vi "UHR-Fleezers Control (host) - 10.4.vi"() -> ()   [LabVIEW 2011] (continued)
  T12 = cluster{"output high":fxp<+/-,16,1>, "output low":fxp<+/-,16,1>}
  T13 = cluster{"Set 1":fxp<+/-,16,1>, "Set 2":fxp<+/-,16,1>}
  T14 = cluster{"proportional gain (Kc)":i16, "integral gain (Kc*Ts/Ti)":i16, "derivative gain (Kc*Td/Ts)":i16}
  T15 = cluster{"Set 1":bool, "Set 2":bool, "Set 3":bool}
  T16 = typedef "LVMinMaxIncTypeDef.ctl" = cluster{"Minimum":dbl, "Maximum":dbl, "Increment":dbl}
  T17 = typedef "Image Type" = u32
  T18 = typedef "nirio_resource_hc.ctl" = tag
  T19 = typedef "openfpgaref.8.6.ctl" = refnum<k20>
  T20 = cluster{"New Image":T2, "New Image":T2, "New Image":T2, "New Image":T2}
  T21 = typedef "XDNodeRunTimeDep.lvlib/timing_clust.ctl" = cluster{"Expected End [f-1]":u64, "Actual End [f-1]":u64, "Finished Late? [f-1]":bool, "Expected End [i-1]":u64, "Actual End [i-1]":u64, "Finished Late? [i-1]":bool, "Expected Start [i]":u64, "Actual Start [i]":u64, "Expected Start [f]":u64, "Actual Start [f]":u64, "Source Name":string, "Structure Name":string, "Period":i64, "Deadline":i64, "Offset":i64, "Start":i64, "Priority":i32, "Timeout":i32, "Mode":T22, "Wakeup Reason":T23, "Error":errorcluster, "Source Type":string, "Secondary Source Type":string, "Global End Time":u64, "Global Start Time":u64, "Frame Duration":u64, "Iteration Duration":u64, "Assigned CPU":i32, "I/O Scan Engine Mode":u32}
  T22 = typedef "XDNodeRunTimeDep.lvlib/nitl_modes.ctl" = enum32{"No Change", "Process missed periods, maintain original phase", "Discard missed periods, maintain original phase", "Process missed periods, ignore original phase", "Discard missed periods, ignore original phase"}
  T23 = typedef "XDNodeRunTimeDep.lvlib/wakeup.ctl" = enum32{"Normal", "Aborted", "Asynchronous wakeup", "Timing source error", "Timed loop error", "Timeout"}
  T24 = enum16{"big-endian, network order", "native, host order", "little-endian"}
  T25 = enum16{"open", "replace", "create", "open or create", "replace or create", "replace or create with confirmation"}
  T26 = cluster{"Scan Range AOD (nm) 2":dbl, "Step Size AOD (nm) 2":dbl, "Scan Speed AOD (nm/s) 2":dbl, "Number of scans (AOD) 2":u16, "Label":string}
  T27 = cluster{"[0]":dbl, "[1]":dbl, "[2]":dbl, "[3]":dbl, "[4]":dbl, "[5]":dbl}
  T28 = cluster{"Diameter (mm)":dbl, "Units":dbl, "Volume":dbl, "Rate":dbl}
  T29 = cluster{"Left":i32, "Top":i32, "Width":u32, "Height":u32}
  T30 = cluster{cluster{"Left":i32, "Top":i32, "Width":u32, "Height":u32}}[]
  T31 = enum32{"setting", "request", "request control", "info", "statistics", "system settings", "I/O sub system", "HRT control", "camera descriptions", "device specific data", "event sub system settings", "event sub system results", "image memory manager"}
  T32 = typedef "AviRefnum.ctl" = refnum<k1>
  T33 = typedef "imagedata.ctl" = cluster{"image type":i32, "image depth":i32, "image":u8[], "mask":u8[], "colors":u32[], "Rectangle":cluster{"left":i16, "top":i16, "right":i16, "bottom":i16}}
  T34 = enum32{"Normal Display", "Dual Display (APD)", "FFT", "High Res Display"}
  T35 = cluster{"Origin Pixel":cluster{"X":sgl, "Y":sgl}, "Angle Relative to Horizontal (deg)":sgl, "Axis Reference":u32}
  T36 = typedef "Simple Grid Descriptor" = cluster{"X Step":sgl, "Y Step":sgl, "Unit":T37}
  T37 = typedef "Image Unit" = enum32{"Undefined", "Angström", "Micrometer", "Millimeter", "Centimeter", "Meter", "Kilometer", "Microinch", "Inch", "Feet", "Nautical miles", "Standard miles", "Steps"}
  T38 = cluster{"averaging mode":u16, "weighting mode":u16, "number of averages":u32}
  T39 = cluster{"dB On (F)":bool, "unwrap phase (F)":bool, "convert to degree (F)":bool}
  T40 = cluster{string, string, string, string, string, string, string, string}
  T41 = cluster{string, string, string, string, string, string, string, string, string, string, string, string}
  T42 = cluster{string, string, string, string, string, string, string, string, string, string, string, string, string}
  T43 = cluster{string, string, string, string, string, string, string, string, string, string, string, string, string, string}
  T44 = cluster{"BD 1 Frequency 1 (MHz)":dbl, "BD 1 Frequency 2 (MHz)":dbl}
  T45 = cluster{"f0":dbl, "df":dbl, "magnitude":dbl[]}[][]
  T46 = cluster{"Green FB Ch 0":i16, "Green FB Ch 1":i16, "Green FB Ch 2":i16}
  T47 = cluster{"Green FB Ch 0":dbl, "Green FB Ch 1":dbl, "Green FB Ch 2":dbl}
diagram:
  w55 = u16 20 items=["1.0"=10, "1.5"=15, "2.0"=20] ("stop bits (10: 1 bit)")
  w62 = T17 2 items=["Grayscale (U8)", "Grayscale (I16)", "Grayscale (SGL)", "Complex (CSG)", "RGB (U32)", "HSL (U32)", "RGB (U64)", "Grayscale (U16)"] ("Image Type")
  w125 = cluster{"output high":i16, "output low":i16} {"output high"=3000, "output low"=0} ("FB output range 1")
  w196 = 10.0 ("y")
  w195 = 32767.0 ("y")
  w211 = 6.0  # clock mult.
  w212 = 49152000.0  # TCXO frequ.
  n1 = Build Array("DIO count 1 (ticks)", "DIO count 2 (ticks)", "DIO count 3 (ticks)") -> (w112:u32[])
  n2 = local read "AO1"() -> (w190:dbl)
  n3 = local read "AO2"() -> (w189:dbl)
  n4 = local read "Scan Increment (MHz)"() -> (w207:dbl)
  n5 = local read "Continuous MCL Scanning"() -> (w177:bool)
  n6 = local read "Fast Scan Dir"() -> (w176:bool)
  n7 = local read "Number of scans (MCL)"() -> (w178:u64)
  n8 = property on="AI Count (ticks)" class="DigNum (strict)"("Val(Sgnl)"="AI Count (ticks)") -> ()  [unwired: 2 in, 2 out]
  n9 = Multiply(x=w190, y=w195) -> (x*y=w192:dbl)
  n10 = Multiply(x=w189, y=w195) -> (x*y=w194:dbl)
  n11 = Divide(x=w192, y=w196) -> (x/y=w191:dbl)
  n12 = Divide(x=w194, y=w196) -> (x/y=w193:dbl)
  n13 = To Word Integer(number=w191) -> (16bit integer=w188:i16)
  n14 = To Word Integer(number=w193) -> (16bit integer=w187:i16)
  n15 = Not(x=w176) -> (.not. x?=w171:bool)
  n16 = local read "Cycles/step (MCL)"() -> (w179:u64)
  n17 = Multiply(x=w207, y=1000.0) -> (x*y=w214:dbl)
  n18 = local read "Scan steps (MCL)"() -> (w180:u64)
  n19 = local write "Trap Pos FIFO Timeout"(u16 0 ("Trap Pos FIFO Timeout")) -> ()
  n20 = local read "Desired Scan Incr (V)"() -> (w182:dbl)
  n21 = Scale By Power Of 2(n=48, x=w214) -> (x*2^n=w215:dbl)
  n22 = Multiply(x=w212, y=w211) -> (x*y=w210:dbl)
  n23 = Divide(x=w215, y=w210) -> (x/y=w209:dbl)
  n24 = local read "Setpoints (V)"() -> (w228:cluster{"Set 1":dbl, "Set 2":dbl})
  n25 = To Quad Integer(1:w209) -> (0:w206:i64)
  n26 = Divide(x=40000000.0, y="AI Count (ticks)") -> (x/y=w167:dbl)
  n27 = Multiply(x=w182, y=32767.0) -> (x*y=w184:dbl)
  n28 = local read "Number Interlace Sets"() -> (w105:u8)
  n29 = Split 1D Array(array=w112, index=w105) -> (first subarray=w114:u32[])  [unwired: 1 out]
  n30 = Add Array Elements(numeric array=w114) -> (sum=w113:u32)
  n31 = local read "# Samples/channel"() -> (w199:u32)
  n32 = local read "Number of F/B Scans (AOD)"() -> (w200:u16)
  n33 = local read "Not-Interlacing Set"() -> (w104:enum32{"Set 1", "Set 2", "Set 3"})
  n34 = To Unsigned Byte Integer(number=w104) -> (unsigned 8bit integer=w110:u8)
  n35 = Index Array(array=w112, index=w110) -> (element=w111:u32)
  n36 = local read "Feedback On/Off"() -> (w231:cluster{"Set 1":bool, "Set 2":bool})
  n37 = local read "PID Gains"() -> (w223:T9)
  n38 = local read "Scan steps (AOD)"() -> (w205:u64)
  n39 = local read "All FB On/Off"() -> (w232:bool)
  n40 = local read "Cycles/step (AOD)"() -> (w204:u64)
  n41 = local write "AI rate (Hz)"(w167) -> ()
  n42 = Divide(x=w184, y=10.0) -> (x/y=w183:dbl)
  n43 = Multiply(x=w205, y=w204) -> (x*y=w203:u64)
  n44 = Multiply(x=3276.7, y=w228) -> (x*y=w227:cluster{"Set 1":dbl, "Set 2":dbl})
  n45 = xnode "Open FPGA VI Reference"("resource name"=T18 "750kHzDAQ") -> ("FPGA VI Reference Out"=w220:T19, "error out"=w219:errorcluster)  [unwired: 1 in]
  n46 = To Word Integer(number=w183) -> (16bit integer=w181:i16)
  n47 = Multiply(x=w203, y=u64 2) -> (x*y=w201:u64)
  n48 = local read "Sets to FIFO (Traps)"() -> (w235:T15)
  n49 = Divide(x=w167, y="FPGA Ave.") -> (x/y=w168:dbl)
  n50 = To Word Integer(number=w227) -> (16bit integer=w226:cluster{"Set 1":i16, "Set 2":i16})
  n51 = Unbundle By Name(w223) -> ("Set 1"=w222:T14, "Set 2"=w221:T14)
  n52 = Multiply(x=w201, y=w200) -> (x*y=w198:u64)
  n53 = local write "Ave. Rate (Hz)"(w168) -> ()
  n54 = Divide(x=w198, y=w199) -> (x/y=w197:dbl)
  n55 = Unbundle By Name(w226) -> ("Set 1"=w225:i16, "Set 2"=w224:i16)
  n56 = local read "2D or 1D Scan"() -> (w126:bool)
  n57 = local write "Data points/scans"(w198) -> ()
  n58 = local read "Scan BD"() -> (w216:bool)
  n59 = And(x=w231, y=w232) -> (x .and. y?=w230:cluster{"Set 1":bool, "Set 2":bool})
  n60 = local write "Data points/scan (f/b)"(w201) -> ()
  n61 = Reciprocal(x=w168) -> (1/x=w169:dbl)
  n62 = local read "N Acq Sets (Traps + Fl.)"() -> (w160:i16)
  n63 = local write "N sets should be saved"(w197) -> ()
  n64 = xnode "Invoke Method"("FPGA VI Reference In"=w220, "error in"=w219) -> ("FPGA VI Reference Out"=w124:T19, "error out"=w134:errorcluster)
  n65 = Unbundle By Name(w230) -> ("Set 1"=w234:bool, "Set 2"=w233:bool)
  n66 = local read "Interlace"() -> (w106:bool)
  n67 = Select(t=w113, s=w106, f=w111) -> (s? t:f=w103:u32)
  n68 = local write "Update Count (MCL)"(w103) -> ()
  n69 = local write "Total Counts (ticks)"(w103) -> ()
  n70 = local write "Ave. Period (s)"(w169) -> ()
  n71 = property on="2D or 1D Scan" class="Bool (strict)"("Val(Sgnl)"=w126) -> ()  [unwired: 2 in, 2 out]
  n72 = local read "GI Frequency, OFF count"() -> (w26:u32)
  n73 = local read "GI Frequency, ON count"() -> (w17:u32)
  n74 = local read "APD Gate OFF Count"() -> (w23:u32)
  n75 = local read "APD Gate ON Count"() -> (w19:u32)
  n76 = xnode "Read/Write Control"("FPGA VI Reference In"=w123, "error in"=w134, "ai count"="AI Count (ticks)", "Interlace ON/OFF"=w106, "Number Interlace Cycles"=w105, "AI1 Sets to FIFO"=w235, "FB On/Off Set 1"=w234, "FB On/Off Set 2"=w233, "Interlace Off Parameters"=w104, "FB Setpoint Set 1"=w225, "FB Setpoint Set 2"=w224, "FB Gains Set 1"=w222, "FB Gains Set 2"=w221, "FB output range 1"=w125, "FB output range 2"=w125, "Cycles per step"=w204, "Scan BD"=w216, "Number of scans"=w200, "Scan steps"=w205, "Scan freq.  increment"=w206, "AO1"=w188, "AO2"=w187, "Scan freq.  increment (MCL)"=w181, "Scan steps (MCL)"=w180, "Cycles per step (MCL)"=w179, "Number of scans (MCL)"=w178, "MCL count"=w103, "Cont. Scan (MCL)"=w177, "MCL Scan Axis"=w171, "1D or 2D Scan?"=w126, "N of AI1 Int Acq Sets"=w160, "Freq or Amp switch first"="Freq or Amp switch first", "Freq switch delay"="Freq switch delay", "Amp switch delay"="Amp switch delay", "Swap F1 and F2"="Swap F1 and F2", "APD to FIFO"=FALSE, "DIO count 1 (ticks)"="DIO count 1 (ticks)", "DIO count 2 (ticks)"="DIO count 2 (ticks)", "DIO count 3 (ticks)"="DIO count 3 (ticks)") -> ("FPGA VI Reference Out"=w30:T19, "error out"=w28:errorcluster)  [unwired: 1 in]
  n77 = local read "On one out of X cycles"() -> (w25:u32)
  n78 = local read "APD Integration Time (s)"() -> (w9:dbl)
  n79 = local read "DMA Update Period (s)"() -> (w8:dbl)
  n80 = Add(x=w19, y=w23) -> (x+y=w21:u32)
  n81 = Add(x=w17, y=w26) -> (x+y=w24:u32)
  n82 = local read "Green Laser ON/Interlacing"() -> (w101:bool)
  n83 = local read "Green laser mode"() -> (w102:enum32{"Laser ON", "Laser OFF", "Interlace"})
  n84 = Multiply(x=w21, y=w25) -> (x*y=w22:u32)
  n85 = Multiply(x=w25, y=w24) -> (x*y=w16:u32)
  n86 = Reciprocal(x=w9) -> (1/x=w6:dbl)
  n87 = Multiply(x=w9, y=40000000.0) -> (x*y=w5:dbl)
  n88 = Divide(x=w8, y=w9) -> (x/y=w11:dbl)
  n89 = Multiply(x="Current When FB OFF (%)", y=655.35) -> (x*y=w89:dbl)
  n90 = local read "Invert APD Gate"() -> (w15:bool)
  n91 = Multiply(x="Green FB Setpoint (mV)", y=3.2767) -> (x*y=w86:dbl)
  n92 = local read "APD Gate"() -> (w14:enum32{"ON", "OFF", "Interlace"})
  n93 = Subtract(x=w22, y=w19) -> (x-y=w20:u32)
  n94 = local write "Green FB Count"(w16) -> ()
  n95 = local write "APD Acq Rate (Hz)"(w6) -> ()
  n96 = To Unsigned Long Integer(number=w5) -> (unsigned 32bit integer=w3:u32)
  n97 = Multiply(x=2.0, y=w11) -> (x*y=w10:dbl)
  n98 = local read "Invert GI"() -> (w98:bool)
  n99 = To Unsigned Word Integer(number=w89) -> (unsigned 16bit integer=w87:u16)
  n100 = Subtract(x=w16, y=w17) -> (x-y=w18:u32)
  n101 = local write "APD Samples/FIFO Acq."(w11) -> ()
  n102 = To Word Integer(number=w86) -> (16bit integer=w84:i16)
  n103 = local write "APD Elements/DMA read"(w10) -> ()
  n104 = case shown="False" w101 {
    tunnel: w102 -> [_ w261]
    tunnel: [enum32{"Laser ON", "Laser OFF", "Interlace"}."Laser OFF" ("Green laser mode") w261] -> w97
    frame False {
    }
    frame True {
    }
  }
  n105 = local write "APD Int. Count"(w3) -> ()
  n106 = local read "Trap Pos. AI1 X Pre-scale"() -> (w41:u16)
  n107 = local read "Trap Pos FB Monitor\nT1 or T2"() -> (w48:bool)
  n108 = local read "Trap Pos FB Int Count"() -> (w34:u16)
  n109 = local read "APD 1 AO Mult."() -> (w13:i16)
  n110 = local read "Trap Pos FB Negate Action"() -> (w47:bool)
  n111 = local read "APD 2 AO Mult."() -> (w12:i16)
  n112 = local read "Trap Pos. FB Offset Factor"() -> (w46:i64)
  n113 = local read "Trap Pos. FB Mult Factor"() -> (w45:i64)
  n114 = local read "Neg. TTrig FPGA"() -> (w2:bool)
  n115 = local read "Trap Pos. FB Gains"() -> (w43:T11)
  n116 = local read "Trap Pos. FB Range"() -> (w44:T12)
  n117 = xnode "Read/Write Control"("FPGA VI Reference In"=w30, "error in"=w28, "Invert APD Gate"=w15, "APD Gate ON Count"=w19, "APD Gate OFF Count"=w20, "APD Acq Rate Count"=w3, "APD Gate Operating Mode"=w14, "APD 1 AO scale factor"=w13, "APD 2 AO scale factor"=w12, "Green interlace ON count"=w17, "Green interlace OFF count"=w18, "Green interlace ON count 2"=w17, "Green interlace OFF count 2"=w18, "Green FB Count"=w16) -> ("FPGA VI Reference Out"=w29:T19, "error out"=w27:errorcluster)
  n118 = xnode "Read/Write Control"("FPGA VI Reference In"=w29, "error in"=w27, "Invert GI 2"=w98, "Operating Mode 2"=w97, "Green FB Gains"="Green FB Gains", "Green FB Setpoint"=w84, "Green FB On/Off"="Green FB On/Off", "Current Out"=w87, "Green int current ON count adj"="Green int current ON count adj", "Operating Mode"=w97, "Invert GI"=w98, "Trap Pos FB Monitor T1 or T2"=w48, "Trap Pos FB Negate Action"=w47, "Trap Pos. FB Offset Factor"=w46, "Trap Pos. FB Mult Factor"=w45, "Trap Pos. FB Range"=w44, "Trap Pos. FB Gains"=w43, "Force feedback"=FALSE, "AI1 X Scale"=w41, "Trap Pos to FIFO"=TRUE, "Trap Pos FB Int Count"=w34, "TTrig Negate Pos"=w2, "FB Trig Integrate"="FB Trig Integrate") -> ("FPGA VI Reference Out"=w99:T19, "error out"=w100:errorcluster)
  n119 = xnode "Invoke Method"("FPGA VI Reference In"=w99, "error in"=w100, "Depth"="Trap AI FIFO Depth") -> ("FPGA VI Reference Out"=w51:T19, "error out"=w50:errorcluster)
  n120 = xnode "Invoke Method"("FPGA VI Reference In"=w51, "error in"=w50, "Depth"="Trap Position FIFO Depth") -> ("FPGA VI Reference Out"=w36:T19, "error out"=w35:errorcluster)
  n121 = flat-sequence {
    tunnel: w124 -> [w266]
    tunnel: [w266] -> w123
    tunnel: [w265] -> w122
    tunnel: [w264] -> w121
    tunnel: [w262] -> w119
    tunnel: [w263] -> w120
    frame #0 {
      w263 = T16 {"Minimum"=0.0, "Maximum"=40.0, "Increment"=1.0} ("Min Max Inc")
      w262 = T16 {"Minimum"=0.0, "Maximum"=50.0, "Increment"=1.0} ("Data Entry Limits")
      w265 = T16 {"Minimum"=60.0, "Maximum"=90.0, "Increment"=1.0} ("Min Max Inc")
      w264 = T16 {"Minimum"=0.0, "Maximum"=50.0, "Increment"=1.0} ("Data Entry Limits")
      n122 = property on="BD 2 Frequency 1 (MHz)" class="DigNum (strict)"("Data Range"=w263) -> ()  [unwired: 2 in, 2 out]
      n123 = property on="BD 2 Frequency 3 (MHz)" class="DigNum (strict)"("Data Range"=w263) -> ()  [unwired: 2 in, 2 out]
      n124 = property on="BD 2 Frequency 2 (MHz)" class="DigNum (strict)"("Data Range"=w263) -> ()  [unwired: 2 in, 2 out]
      n125 = property on="BD 1 Frequency 1 (MHz)" class="DigNum (strict)"("Data Range"=w265) -> ()  [unwired: 2 in, 2 out]
      n126 = property on="BD 1 Frequency 2 (MHz)" class="DigNum (strict)"("Data Range"=w265) -> ()  [unwired: 2 in, 2 out]
      n127 = property on="BD 1 Frequency 3 (MHz)" class="DigNum (strict)"("Data Range"=w265) -> ()  [unwired: 2 in, 2 out]
      n128 = property on="BD 2 Amplitude 1 (%)" class="DigNum (strict)"("Data Range"=w262) -> ()  [unwired: 2 in, 2 out]
      n129 = property on="BD 2 Amplitude 2 (%)" class="DigNum (strict)"("Data Range"=w262) -> ()  [unwired: 2 in, 2 out]
      n130 = property on="BD 2 Amplitude 3 (%)" class="DigNum (strict)"("Data Range"=w262) -> ()  [unwired: 2 in, 2 out]
      n131 = property on="BD 1 Amplitude 3 (%)" class="DigNum (strict)"("Data Range"=w264) -> ()  [unwired: 2 in, 2 out]
      n132 = property on="BD 1 Amplitude 2 (%)" class="DigNum (strict)"("Data Range"=w264) -> ()  [unwired: 2 in, 2 out]
      n133 = property on="BD 1 Amplitude 1 (%)" class="DigNum (strict)"("Data Range"=w264) -> ()  [unwired: 2 in, 2 out]
      "X RF Frequency Limits (MHz)" <- w265
      "X RF Amplitude Limits (%)" <- w264
      "Y RF Amplitude Limits (%)" <- w262
      "Y RF Frequency Limits (MHz)" <- w263
    }
  }
  n134 = xnode "Invoke Method"("FPGA VI Reference In"=w36, "error in"=w35) -> ("FPGA VI Reference Out"=w133:T19, "error out"=w132:errorcluster)  [unwired: 1 out]
  n135 = flat-sequence "Initial FPGA Loop Relative Phase Adjustment" {
    tunnel: "Initial Phase Adjustment (AI1)" -> [w277]
    tunnel: "Initial Phase Adjustment (GI)" -> [w276]
    tunnel: w133 -> [w275]
    tunnel: w132 -> [w274]
    tunnel: "Initial Phase Adj. (MCL)" -> [w273]
    tunnel: [w278] -> w142
    tunnel: [w272] -> w138
    tunnel: "Initial Phase Adjustment (APD Acq)" -> [w271]
    tunnel: "Initial Phase Adjustment (APD 1 Gate)" -> [w270]
    tunnel: "Initial Phase Adjustment (Green FB)" -> [w269]
    tunnel: "Initial Phase Adjustment (GI) 2" -> [w268]
    tunnel: "Initial Phase Adjustment (APD 2 Gate)" -> [w267]
    tunnel: w142 -> [w280]
    tunnel: [w281] -> w139
    tunnel: w138 -> [w281]
    tunnel: [w280] -> w137
    tunnel: w139 -> [w284]
    tunnel: w137 -> [w283]
    tunnel: [w286] -> w136
    tunnel: [w285] -> w135
    tunnel: [w288] -> w140
    tunnel: [w289] -> w141
    tunnel: w136 -> [w289]
    tunnel: w135 -> [w288]
    frame #0 {
      n136 = xnode "Read/Write Control"("FPGA VI Reference In"=w275, "error in"=w274, "Phase count adjustment"=w277, "Phase count adjustment (GI)"=w276, "Phase count adjustment (MCL)"=w273, "Phase Count Adjustment (APD Acq)"=w271, "Phase count adjustment (APD 1 Gate)"=w270, "Phase count adjustment (APD 2 Gate)"=w267, "Phase count adjustment (Green FB)"=w269, "Phase count adjustment (GI) 2"=w268) -> ("FPGA VI Reference Out"=w272:T19, "error out"=w278:errorcluster)
    }
    frame #1 {
      n137 = Wait (ms)(milliseconds to wait=u32 100) -> ()  [unwired: 1 out]
    }
    frame #2 {
      w282 = TRUE
      n138 = xnode "Read/Write Control"("FPGA VI Reference In"=w284, "error in"=w283, "+ phase"=w282, "+ phase (GI)"=w282, "+ phase (MCL)"=w282, "+ phase (APD Acq)"=w282, "+ phase (APD 1 Gate)"=w282, "+ phase (APD 2 Gate)"=w282, "+ phase (Green FB)"=w282, "+ phase (GI) 2"=w282) -> ("FPGA VI Reference Out"=w285:T19, "error out"=w286:errorcluster)
    }
    frame #3 {
      n139 = Wait (ms)(milliseconds to wait=u32 100) -> ()  [unwired: 1 out]
    }
  }
  n140 = local read "Phase adj. (Green FB)"() -> (w115:i16)
  n141 = local read "Phase adj. (GI) 2"() -> (w90:i16)
  n142 = local read "Phase adjust (MCL)"() -> (w172:i16)
  n143 = local read "Phase adj. (AI1)"() -> (w174:i16)
  n144 = local read "Phase adj. (GI)"() -> (w173:i16)
  n145 = xnode "Read/Write Control"("FPGA VI Reference In"=w140, "error in"=w141, "Phase count adjustment"=w174, "Phase count adjustment (GI)"=w173, "Phase count adjustment (MCL)"=w172, "Phase Count Adjustment (APD Acq)"="Phase Adj. (APD Acq)", "Phase count adjustment (APD 1 Gate)"="Phase Adj. (APD 1 Gate)", "Phase count adjustment (APD 2 Gate)"="Phase Adj. (APD 2 Gate)", "Phase count adjustment (Green FB)"=w115, "Phase count adjustment (GI) 2"=w90) -> ("FPGA VI Reference Out"=w76:T19, "error out"=w149:errorcluster)
  n146 = call "Initialize RF boards - interlace 3.vi"("error in"=w149, "FPGA VI Reference In"=w76) -> ("error out"=w147:errorcluster, "FPGA VI Reference Out"=w148:T19)
  n147 = call "set RF board frequency - interlace.vi"("Board 2 Frequency Limits"=w120, "Board 1 Frequency Limits"=w122, "error in"=w147, "FPGA VI Reference In"=w148, "Board 2 Frequency 3 (MHz)"="BD 2 Frequency 3 (MHz)", "Board 1 Frequency 3 (MHz)"="BD 1 Frequency 3 (MHz)", "Board 2 Frequency 2 (MHz)"="BD 2 Frequency 2 (MHz)", "Board 2 Frequency 1 (MHz)"="BD 2 Frequency 1 (MHz)", "Board 1 Frequency 2 (MHz)"="BD 1 Frequency 2 (MHz)", "Board 1 Frequency 1  (MHz)"="BD 1 Frequency 1 (MHz)") -> ("error out"=w250:errorcluster, "FPGA VI Reference Out"=w251:T19)
  n148 = call "set RF board amplitude - interlace.vi"("Board 2 Amplitude Limits"=w119, "Board 1 Amplitude Limits"=w121, "error in"=w250, "FPGA VI Reference In"=w251, "Board 2 Amplitude 3 (%)"="BD 2 Amplitude 3 (%)", "Board 1 Amplitude 3 (%)"="BD 1 Amplitude 3 (%)", "Board 2 Amplitude 2 (%)"="BD 2 Amplitude 2 (%)", "Board 2 Amplitude 1 (%)"="BD 2 Amplitude 1 (%)", "Board 1 Amplitude 2 (%)"="BD 1 Amplitude 2 (%)", "Board 1 Amplitude 1 (%)"="BD 1 Amplitude 1 (%)") -> ("error out"=w238:errorcluster, "FPGA VI Reference Out"=w239:T19)
  n149 = flat-sequence {
    tunnel: w239 -> [w298]
    tunnel: w238 -> [w297]
    tunnel: [w296] -> w243
    tunnel: [w295] -> w242
    tunnel: [w302] -> w241
    tunnel: w243 -> [w302]
    tunnel: [w301] -> w240
    tunnel: w242 -> [w301]
    tunnel: w241 -> [w311]
    tunnel: w240 -> [w310]
    tunnel: [w309] -> w38
    tunnel: [w308] -> w37
    frame #0 {
      n150 = local read "Trap 1 (ON/OFF)"() -> (w290:bool)
      n151 = xnode "Read/Write Control"("FPGA VI Reference In"=w298, "error in"=w297, "Direct RF Box  Communication"=FALSE) -> ("FPGA VI Reference Out"=w296:T19, "error out"=w295:errorcluster)
      n152 = local write "Saving..."(FALSE ("Saving Data")) -> ()
      n153 = local write "Stop All"(FALSE ("Stop All")) -> ()
      n154 = local write "Index"(1.0 ("Index")) -> ()
      n155 = property on="Trap 1 ON" class="Bool (strict)"("Value"=w290) -> ()  [unwired: 2 in, 2 out]
      "Manipulating Trap" <- FALSE ("Manipulating Trap")
    }
    frame #1 {
      n156 = local read "Trap 2 (ON/OFF)"() -> (w300:bool)
      n157 = Wait (ms)(milliseconds to wait=u32 10) -> ()  [unwired: 1 out]
      n158 = property on="Trap 2 ON" class="Bool (strict)"("Val(Sgnl)"=w300) -> ()  [unwired: 2 in, 2 out]
    }
    frame #2 {
      n159 = local read "Scan Range (nm)"() -> (w304:dbl)
      n160 = xnode "Read/Write Control"("FPGA VI Reference In"=w311, "error in"=w310, "FPGA Controls  RF Box"=TRUE ("Direct RF Box  Communication")) -> ("FPGA VI Reference Out"=w309:T19, "error out"=w308:errorcluster)
      n161 = call "Update messages.vi"("Message to add"="UHR-Fleezers ready.", "Old message string"="") -> ("New message string"=w307:string)
      n162 = local write "Messages"(w307) -> ()
      n163 = property on="Scan Range (nm)" class="DigNum (strict)"("Val(Sgnl)"=w304) -> ()  [unwired: 2 in, 2 out]
    }
  }
  n164 = Subtract(x="BD 1 Frequency 1 (MHz)", y="BD 1 Frequency 2 (MHz)") -> (x-y=w159:dbl)
  n165 = Subtract(x="BD 2 Frequency 1 (MHz)", y="BD 2 Frequency 2 (MHz)") -> (x-y=w158:dbl)
  n166 = Square(x=w158) -> (x^2=w156:dbl)
  n167 = Square(x=w159) -> (x^2=w157:dbl)
  n168 = Add(x=w157, y=w156) -> (x+y=w155:dbl)
  n169 = Square Root(x=w155) -> (sqrt(x)=w154:dbl)
  n170 = local write "Trap Delta (MHz)"(w154) -> ()
  n171 = call "IMAQ Create"("Image Name"="APD 1 Image", "Image Type"=w62) -> ("New Image"=w61:T2)  [unwired: 3 in, 1 out]
  n172 = call "IMAQ Create"("Image Name"="APD 2 Image", "Image Type"=w62) -> ("New Image"=w60:T2)  [unwired: 3 in, 1 out]
  n173 = call "IMAQ Create"("Image Name"="Det. X Image", "Image Type"=w62) -> ("New Image"=w59:T2)  [unwired: 3 in, 1 out]
  n174 = call "IMAQ Create"("Image Name"="Det. Y Image", "Image Type"=w62) -> ("New Image"=w58:T2)  [unwired: 3 in, 1 out]
  n175 = Bundle("New Image"=w61, "New Image"=w60, "New Image"=w59, "New Image"=w58) -> (w57:T20)  [unwired: 1 in]
  n176 = call-poly "VISA Configure Serial Port"("VISA resource name"="Sample Chamber Stage Serial Port") -> ("VISA resource name out"=w71:refnum<visa-resource-name>, "error out"=w72:errorcluster)  [unwired: 5 in, 8 out]
  "Stage Control Serial Error" <- w72
  n177 = call-poly "VISA Configure Serial Port"("VISA resource name"="Harvard Syringe Pump Serial Port", "baud rate (9600)"=u32 115200, "stop bits (10: 1 bit)"=w55) -> ("VISA resource name out"=w52:refnum<visa-resource-name>, "error out"=w53:errorcluster)  [unwired: 4 in, 7 out]
  n178 = node-c288() -> (w67:T21)  [unwired: 4 in]
  n179 = timed-loop "Run Scripts, including: stage motion" {
    tunnel: w72 -> [w315]
    tunnel: w71 -> [w316]
    tunnel: [w316] -> w70
    tunnel: [w315] -> w69
    timing: w67 -> [_]
    timing-out: [_] -> w66
    tunnel: w52 -> [w314]
    tunnel: w53 -> [w313]
    stop <- w317 stop-if-true
    n180 = node-c288() -> ()  [unwired: 1 in, 1 out]
    n181 = event shown="[7] \"Dip for Protein\": Value Change" {
      selector: _ -> [_ _ _ _ _ _ _ _ _ _ _ _ _ _ _ _ _ _]
      dyn-events: _ -> [_ _ _ _ _ _ _ _ _ _ _ _ _ _ _ _ _ _]
      timeout: _ -> [_ _ _ _ _ _ _ _ _ _ _ _ _ _ _ _ _ _]
      tunnel: ["Set Position" "Move to Position" "Move Cap. 1 (DNA Bottom)" "Move Cap. 2 (ADig Top)" _ "Cal/Data Acq. Spot" "Dump Beads" _ _ _ "Got ADig bead" "Take Force FB Data\nScript" "Test move stage" "Got DNA bead" "Take Stepping Data" _ "Take Detection Laser\nImage" _] -> _
      tunnel: [_ _ _ _ _ _ _ _ _ _ _ _ _ _ _ _ _ w894] -> w317
      tunnel: w315 -> [w335 w343 w357 w395 w424 w464 w552 w581 w684 w710 _ w747 w792 _ _ _ _ _]
      tunnel: w316 -> [w336 w344 w358 w396 w425 w465 w553 w582 w685 w711 _ w748 w793 _ _ _ _ _]
      tunnel: w314 -> [_ _ _ _ _ _ _ _ _ _ _ _ _ _ _ _ _ _]
      tunnel: w313 -> [_ _ _ _ _ _ _ _ _ _ _ _ _ _ _ _ _ _]
      event "Set Position", "Set Position 2", "Set Position 3", "Set Position 4", "Set Position 5", "Set Position 1": Value Change {
        n182 = event-data() -> ()  [unwired: 1 in, 5 out]
        n183 = Build Array("Set Position 1", "Set Position 2", "Set Position 3", "Set Position 4", "Set Position 5") -> (w334:bool[])
        n184 = Boolean Array To Number(Boolean array=w334) -> (number=w333:u32)
        n185 = Logarithm Base 2(1:w333) -> (0:w325:dbl)
        n186 = call "Read Stage Position.vi"("error in"=w335, "VISA resource name in"=w336) -> ("Current Position"=w340:cluster{dbl, dbl, dbl}, "error out"=w339:errorcluster)  [unwired: 2 out]
        n187 = Decrement(x="Position") -> (x-1=w323:dbl)
        n188 = Greater Or Equal?(x=w325, y=0.0) -> (x >= y?=w326:bool)
        n189 = Cluster To Array(cluster=w340) -> (array=w337:dbl[])
        n190 = local write "Stage Control Serial Error"(w339) -> ()
        n191 = Select(t=w325, s=w326, f=w323) -> (s? t:f=w322:dbl)
        n192 = Increment(x=w322) -> (x+1=w321:dbl)
        n193 = Build Array (concatenate)(w321, w337) -> (w320:dbl[])
        n194 = Replace Array Subset(array="Saved Stage Positions", new element=w320, index (row)=w322) -> (w338:dbl[][])  [unwired: 1 in]
        n195 = local write "Saved Stage Positions"(w338) -> ()
      }
      event "Move to Position": Value Change {
        n196 = event-data() -> ()  [unwired: 1 in, 5 out]
        n197 = flat-sequence {
          tunnel: w344 -> [w348]
          tunnel: w343 -> [w347]
          frame #0 {
            n198 = local read "Saved Stage Positions"() -> (w350:dbl[][])
            n199 = local read "Position"() -> (w349:dbl)
            n200 = local write "Stage Moving"(TRUE ("Stage Moving")) -> ()
            n201 = call "move to saved stage position.vi"("error in"=w347, "Stage VISA resource name in"=w348, "Position"=w349, "Saved Stage Positions"=w350) -> ("error out"=w346:errorcluster)  [unwired: 1 out]
            n202 = local write "Stage Control Serial Error"(w346) -> ()
          }
          frame #1 {
            n203 = call <vilib>:"Beep.vi"() -> ()  [unwired: 3 in, 9 out]
            n204 = local write "Stage Moving"(FALSE ("Stage Moving")) -> ()
          }
        }
      }
      event "Move Cap. 1 (DNA Bottom)": Value Change {
        n205 = event-data() -> ()  [unwired: 1 in, 5 out]
        n206 = local write "Move Cap. 1 (DNA Bottom)"(FALSE ("Move Cap. 1 (DNA Right)")) -> ()
        n207 = flat-sequence {
          tunnel: w357 -> [w364]
          tunnel: w358 -> [w365]
          tunnel: [w365] -> w355
          tunnel: [w364] -> w354
          tunnel: "Cap 1 Samp Flow ON" -> [w362]
          tunnel: w355 -> [w368]
          tunnel: w354 -> [w367]
          tunnel: "Cap 1 Samp Flow ON" -> [w381]
          frame #0 {
            n208 = local read "Sample Channel\nFlow"() -> (w363:bool)
            n209 = Not(x=w363) -> (.not. x?=w361:bool)
            n210 = And(x=w362, y=w361) -> (x .and. y?=w360:bool)
            n211 = case shown="True" w360 {
              frame False {
              }
              frame True {
                n212 = property on="Sample Channel\nFlow" class="Bool (strict)"("Val(Sgnl)"=TRUE ("Value (Signaling)")) -> ()  [unwired: 2 in, 2 out]
              }
            }
          }
          frame #1 {
            n213 = local read "Saved Stage Positions"() -> (w378:dbl[][])
            n214 = Array Subset(array=w378, index (row)=0 ("index"), length (row)=1 ("length"), index (col)=1 ("index"), length (col)=3 ("length")) -> (w375:dbl[][])
            n215 = local write "Stage Moving"(TRUE ("Stage Moving")) -> ()
            n216 = Reshape Array(w375, 3 ("dimension size")) -> (w373:dbl[])
            n217 = Array To Cluster(array=w373) -> (cluster=w372:cluster{"[0]":dbl, "[1]":dbl, "[2]":dbl})
            n218 = call "Set Stage Position.vi"("Position"=w372, "error in"=w367, "VISA resource name in"=w368) -> ("error out"=w371:errorcluster)  [unwired: 2 out]
            n219 = local write "Stage Control Serial Error"(w371) -> ()
          }
          frame #2 {
            n220 = local read "Sample Channel\nFlow"() -> (w382:bool)
            n221 = local write "Stage Moving"(FALSE ("Stage Moving")) -> ()
            n222 = call <vilib>:"Beep.vi"() -> ()  [unwired: 3 in, 9 out]
            n223 = And(x=w381, y=w382) -> (x .and. y?=w380:bool)
            n224 = case shown="True" w380 {
              frame False {
              }
              frame True {
                n225 = property on="Sample Channel\nFlow" class="Bool (strict)"("Val(Sgnl)"=FALSE ("Value (Signaling)")) -> ()  [unwired: 2 in, 2 out]
              }
            }
          }
          frame #3 {
            n226 = case shown="True" "Cap 1 Flow ON" {
              frame False {
              }
              frame True {
                n227 = property on="Inject Pump 1" class="Bool (strict)"("Val(Sgnl)"=TRUE ("Value (Signaling)")) -> ()  [unwired: 2 in, 2 out]
              }
            }
            n228 = case shown="True" TRUE {
              tunnel: "Cap 1 T ON" -> [w389 w390]
              frame False {
                n229 = property on="Trap 1 (ON/OFF)" class="Bool (strict)"("Val(Sgnl)"=w389) -> ()  [unwired: 2 in, 2 out]
              }
              frame True {
                n230 = property on="Trap 2 (ON/OFF)" class="Bool (strict)"("Val(Sgnl)"=w390) -> ()  [unwired: 2 in, 2 out]
              }
            }
          }
        }
      }
      event "Move Cap. 2 (ADig Top)": Value Change {
        n231 = event-data() -> ()  [unwired: 1 in, 5 out]
        n232 = local write "Move Cap. 2 (ADig Top)"(FALSE ("Move Cap. 2 (ADig Left)")) -> ()
        n233 = flat-sequence {
          tunnel: w395 -> [w399]
          tunnel: w396 -> [w400]
          tunnel: [w400] -> w393
          tunnel: [w399] -> w392
          tunnel: "Cap 2 Samp Flow ON" -> [w398]
          tunnel: w393 -> [w403]
          tunnel: w392 -> [w402]
          tunnel: "Cap 2 Samp Flow ON" -> [w415]
          frame #0 {
            n234 = case shown="True" w398 {
              frame False {
              }
              frame True {
                n235 = property on="Sample Channel\nFlow" class="Bool (strict)"("Val(Sgnl)"=TRUE ("Value (Signaling)")) -> ()  [unwired: 2 in, 2 out]
              }
            }
          }
          frame #1 {
            n236 = local read "Saved Stage Positions"() -> (w413:dbl[][])
            n237 = local write "Stage Moving"(TRUE ("Stage Moving")) -> ()
            n238 = Array Subset(array=w413, index (row)=1 ("index"), length (row)=1 ("length"), index (col)=1 ("index"), length (col)=3 ("length")) -> (w410:dbl[][])
            n239 = Reshape Array(w410, 3 ("dimension size")) -> (w408:dbl[])
            n240 = Array To Cluster(array=w408) -> (cluster=w407:cluster{"[0]":dbl, "[1]":dbl, "[2]":dbl})
            n241 = call "Set Stage Position.vi"("Position"=w407, "error in"=w402, "VISA resource name in"=w403) -> ("error out"=w406:errorcluster)  [unwired: 2 out]
            n242 = local write "Stage Control Serial Error"(w406) -> ()
          }
          frame #2 {
            n243 = case shown="True" w415 {
              frame False {
              }
              frame True {
                n244 = property on="Sample Channel\nFlow" class="Bool (strict)"("Val(Sgnl)"=FALSE ("Value (Signaling)")) -> ()  [unwired: 2 in, 2 out]
              }
            }
            n245 = local write "Stage Moving"(FALSE ("Stage Moving")) -> ()
            n246 = call <vilib>:"Beep.vi"() -> ()  [unwired: 3 in, 9 out]
          }
          frame #3 {
            n247 = case shown="True" "Cap 2 Flow ON" {
              frame False {
              }
              frame True {
                n248 = property on="Inject Pump 3" class="Bool (strict)"("Val(Sgnl)"=TRUE ("Value (Signaling)")) -> ()  [unwired: 2 in, 2 out]
              }
            }
            n249 = case shown="True" TRUE {
              tunnel: "Cap 2 T ON" -> [w422 w423]
              frame False {
                n250 = property on="Trap 2 (ON/OFF)" class="Bool (strict)"("Val(Sgnl)"=w422) -> ()  [unwired: 2 in, 2 out]
              }
              frame True {
                n251 = property on="Trap 1 (ON/OFF)" class="Bool (strict)"("Val(Sgnl)"=w423) -> ()  [unwired: 2 in, 2 out]
              }
            }
          }
        }
      }
      event "+z", "-z": Value Change {
        n252 = event-data() -> ()  [unwired: 1 in, 5 out]
        n253 = flat-sequence {
          tunnel: w424 -> [w446]
          tunnel: w425 -> [w426]
          frame #0 {
            n254 = call "Read Stage Position.vi"("error in"=w446, "VISA resource name in"=w426) -> ("Current Position"=w431:cluster{dbl, dbl, dbl}, "error out"=w444:errorcluster, "VISA resource name out"=w445:refnum<visa-resource-name>)  [unwired: 1 out]
            n255 = local read "Saved Stage Positions"() -> (w455:dbl[][])
            n256 = Divide(x="z nudge increment (um)", y=1000.0) -> (x/y=w443:dbl)
            n257 = Boolean To (0,1)(Boolean="+z") -> (0, 1=w435:i16)
            n258 = Boolean To (0,1)(Boolean="-z") -> (0, 1=w436:i16)
            n259 = Array Subset(array=w455, index (row)=1 ("index"), length (row)=1 ("length"), index (col)=1 ("index"), length (col)=3 ("length")) -> (w452:dbl[][])
            n260 = Multiply(x=w435, y=w443) -> (x*y=w439:dbl)
            n261 = Multiply(x=w436, y=w443) -> (x*y=w437:dbl)
            n262 = Unbundle(w431) -> (w429:dbl, w428:dbl, w432:dbl)
            n263 = Negate(x=w437) -> (-x=w438:dbl)
            n264 = Reshape Array(w452, 3 ("dimension size")) -> (w450:dbl[])
            n265 = Add(x=w439, y=w438) -> (x+y=w440:dbl)
            n266 = Array To Cluster(array=w450) -> ()  [unwired: 1 out]
            n267 = Add(x=w440, y=w432) -> (x+y=w430:dbl)
            n268 = Bundle(cluster=w431, w429, w428, w430) -> (w427:cluster{dbl, dbl, dbl})
            n269 = call "Set Stage Position.vi"("Position"=w427, "error in"=w444, "VISA resource name in"=w445) -> ("error out"=w449:errorcluster)  [unwired: 2 out]
            n270 = local write "Stage Moving"(TRUE ("Stage Moving")) -> ()
            n271 = local write "Stage Control Serial Error"(w449) -> ()
          }
          frame #1 {
            n272 = local write "Stage Moving"(FALSE ("Stage Moving")) -> ()
            n273 = call <vilib>:"Beep.vi"() -> ()  [unwired: 3 in, 9 out]
          }
        }
      }
      event "Cal/Data Acq. Spot": Value Change {
        n274 = event-data() -> ()  [unwired: 1 in, 5 out]
        n275 = flat-sequence {
          tunnel: w464 -> [w472]
          tunnel: w465 -> [w473]
          tunnel: [w473] -> w461
          tunnel: [w472] -> w460
          tunnel: "Daq spot flow on" -> [w470]
          tunnel: w461 -> [w478]
          tunnel: w460 -> [w477]
          tunnel: ["Cal @ (MHz)"] -> w462
          tunnel: "Daq spot flow on" -> [w483]
          tunnel: w462 -> [w494]
          tunnel: ["W/ Offset 1"] -> w458
          tunnel: w462 -> [w515]
          tunnel: w458 -> [w513]
          frame #0 {
            n276 = local read "Sample Channel\nFlow"() -> (w469:bool)
            n277 = Not(x=w469) -> (.not. x?=w468:bool)
            n278 = And(x=w470, y=w468) -> (x .and. y?=w467:bool)
            n279 = case shown="True" w467 {
              frame False {
              }
              frame True {
                n280 = property on="Sample Channel\nFlow" class="Bool (strict)"("Val(Sgnl)"=TRUE ("Value (Signaling)")) -> ()  [unwired: 2 in, 2 out]
              }
            }
            n281 = Wait (ms)(milliseconds to wait=u32 250) -> ()  [unwired: 1 out]
          }
          frame #1 {
            n282 = local read "Saved Stage Positions"() -> (w475:dbl[][])
            n283 = local write "Stage Moving"(TRUE ("Stage Moving")) -> ()
            n284 = call "move to saved stage position.vi"("error in"=w477, "Stage VISA resource name in"=w478, "Position"="Cal Stage Position", "Saved Stage Positions"=w475) -> ("error out"=w476:errorcluster)  [unwired: 1 out]
            n285 = local write "Stage Control Serial Error"(w476) -> ()
          }
          frame #2 {
            n286 = property on="Trap Delta (MHz)" class="DigNum (strict)"("Val(Sgnl)"="Cal @ (MHz)") -> ()  [unwired: 2 in, 2 out]
            n287 = local read "Sample Channel\nFlow"() -> (w482:bool)
            n288 = local write "Stage Moving"(FALSE ("Stage Moving")) -> ()
            n289 = call <vilib>:"Beep.vi"() -> ()  [unwired: 3 in, 9 out]
            n290 = And(x=w483, y=w482) -> (x .and. y?=w481:bool)
            n291 = case shown="True" w481 {
              frame False {
              }
              frame True {
                n292 = property on="Sample Channel\nFlow" class="Bool (strict)"("Val(Sgnl)"=FALSE ("Value (Signaling)")) -> ()  [unwired: 2 in, 2 out]
              }
            }
          }
          frame #3 {
            n293 = Wait (ms)(milliseconds to wait=u32 500) -> ()  [unwired: 1 out]
          }
          frame #4 {
            n294 = property on="Save Calibration" class="Bool (strict)"("Val(Sgnl)"=TRUE ("Value (Signaling)")) -> ()  [unwired: 2 in, 2 out]
          }
          frame #5 {
            n295 = Wait (ms)(milliseconds to wait=u32 4000) -> ()  [unwired: 1 out]
          }
          frame #6 {
            n296 = while {
              stop <- w490 stop-if-true
              n297 = local read "Saving..."() -> (w491:bool)
              n298 = Wait (ms)(milliseconds to wait=u32 100) -> ()  [unwired: 1 out]
              n299 = Not(x=w491) -> (.not. x?=w490:bool)
            }
          }
          frame #7 {
            n300 = case shown="False" "W/ Offset 1" {
              tunnel: w494 -> [_ w495]
              frame False {
              }
              frame True {
                n301 = stacked-sequence {
                  tunnel: w495 -> [_ _ _ _ _ _ _ w512]
                  frame #0 {
                    n302 = property on="Trap Delta (MHz)" class="DigNum (strict)"("Val(Sgnl)"="Offset 1 Start (MHz)") -> ()  [unwired: 2 in, 2 out]
                    n303 = Replace Array Subset(array=u32[] [0] ("Index Values"), new element="Offset 1 Set", index=0) -> (w496:u32[])
                    n304 = property on="Saved AOD Raster Scan Parameter Sets" class="Arr (strict)"("Index Values"=w496) -> ()  [unwired: 2 in, 2 out]
                  }
                  frame #1 {
                    n305 = Wait (ms)(milliseconds to wait=u32 200) -> ()  [unwired: 1 out]
                  }
                  frame #2 {
                    n306 = property on="Load parameters" class="Bool (strict)"("Val(Sgnl)"=TRUE ("Value (Signaling)")) -> ()  [unwired: 2 in, 2 out]
                  }
                  frame #3 {
                    n307 = Wait (ms)(milliseconds to wait=u32 200) -> ()  [unwired: 1 out]
                  }
                  frame #4 {
                    n308 = property on="Trap Raster Scan" class="Bool (strict)"("Val(Sgnl)"=TRUE ("Value (Signaling)")) -> ()  [unwired: 2 in, 2 out]
                  }
                  frame #5 {
                    n309 = Wait (ms)(milliseconds to wait=u32 2000) -> ()  [unwired: 1 out]
                  }
                  frame #6 {
                    n310 = while {
                      stop <- w509 stop-if-true
                      n311 = local read "Raster Scanning..."() -> (w511:bool)
                      n312 = local read "Saving..."() -> (w507:bool)
                      n313 = Wait (ms)(milliseconds to wait=u32 100) -> ()  [unwired: 1 out]
                      n314 = Not(x=w507) -> (.not. x?=w506:bool)
                      n315 = Not(x=w511) -> (.not. x?=w508:bool)
                      n316 = And(x=w508, y=w506) -> (x .and. y?=w509:bool)
                    }
                  }
                  frame #7 {
                    n317 = property on="Trap Delta (MHz)" class="DigNum (strict)"("Val(Sgnl)"=w512) -> ()  [unwired: 2 in, 2 out]
                  }
                }
              }
            }
          }
          frame #8 {
            n318 = local read "Save ave N"() -> (w514:dbl)
            n319 = case shown="False" "W/ Offset 2" {
              tunnel: w515 -> [_ w522]
              tunnel: w514 -> [_ w521]
              tunnel: w513 -> [w517 _]
              frame False {
                n320 = case shown="False" w517 {
                  frame False {
                    n321 = Multiply(x="Cal read wait (s)", y=u32 1000 ("milliseconds to wait")) -> (x*y=w519:u32)
                    n322 = Wait (ms)(milliseconds to wait=w519) -> ()  [unwired: 1 out]
                  }
                  frame True {
                  }
                }
              }
              frame True {
                n323 = stacked-sequence {
                  tunnel: w522 -> [_ _ _ _ _ _ _ _ _ w543 _ _]
                  tunnel: w521 -> [_ _ _ _ _ _ _ _ _ w541 _ _]
                  frame #0 {
                    n324 = property on="Save ave N" class="DigNum (strict)"("Val(Sgnl)"=1.0 ("Value (Signaling)")) -> ()  [unwired: 2 in, 2 out]
                  }
                  frame #1 {
                    n325 = Wait (ms)(milliseconds to wait=u32 500) -> ()  [unwired: 1 out]
                  }
                  frame #2 {
                    n326 = property on="Trap Delta (MHz)" class="DigNum (strict)"("Val(Sgnl)"="Offset 2 Start (MHz)") -> ()  [unwired: 2 in, 2 out]
                    n327 = Replace Array Subset(array=u32[] [0] ("Index Values"), new element="Offset 2 Set", index=0) -> (w527:u32[])
                    n328 = property on="Saved AOD Raster Scan Parameter Sets" class="Arr (strict)"("Index Values"=w527) -> ()  [unwired: 2 in, 2 out]
                  }
                  frame #3 {
                    n329 = Wait (ms)(milliseconds to wait=u32 500) -> ()  [unwired: 1 out]
                  }
                  frame #4 {
                    n330 = property on="Load parameters" class="Bool (strict)"("Val(Sgnl)"=TRUE ("Value (Signaling)")) -> ()  [unwired: 2 in, 2 out]
                  }
                  frame #5 {
                    n331 = Wait (ms)(milliseconds to wait=u32 500) -> ()  [unwired: 1 out]
                  }
                  frame #6 {
                    n332 = property on="Trap Raster Scan" class="Bool (strict)"("Val(Sgnl)"=TRUE ("Value (Signaling)")) -> ()  [unwired: 2 in, 2 out]
                  }
                  frame #7 {
                    n333 = Wait (ms)(milliseconds to wait=u32 2000) -> ()  [unwired: 1 out]
                  }
                  frame #8 {
                    n334 = while {
                      stop <- w536 stop-if-true
                      n335 = local read "Raster Scanning..."() -> (w539:bool)
                      n336 = local read "Saving..."() -> (w537:bool)
                      n337 = Wait (ms)(milliseconds to wait=u32 100) -> ()  [unwired: 1 out]
                      n338 = Not(x=w537) -> (.not. x?=w535:bool)
                      n339 = Not(x=w539) -> (.not. x?=w538:bool)
                      n340 = And(x=w538, y=w535) -> (x .and. y?=w536:bool)
                    }
                  }
                  frame #9 {
                    n341 = property on="Trap Delta (MHz)" class="DigNum (strict)"("Val(Sgnl)"=w543) -> ()  [unwired: 2 in, 2 out]
                    n342 = property on="Saved AOD Raster Scan Parameter Sets" class="Arr (strict)"("Index Values"=u32[] [0]) -> ()  [unwired: 2 in, 2 out]
                    n343 = property on="Save ave N" class="DigNum (strict)"("Val(Sgnl)"=w541) -> ()  [unwired: 2 in, 2 out]
                  }
                  frame #10 {
                    n344 = Wait (ms)(milliseconds to wait=u32 500) -> ()  [unwired: 1 out]
                  }
                  frame #11 {
                    n345 = property on="Load parameters" class="Bool (strict)"("Val(Sgnl)"=TRUE ("Value (Signaling)")) -> ()  [unwired: 2 in, 2 out]
                  }
                }
              }
            }
          }
          frame #9 {
            n346 = property on="Read Cal" class="Bool (strict)"("Val(Sgnl)"=TRUE ("Value (Signaling)")) -> ()  [unwired: 2 in, 2 out]
          }
          frame #10 {
            n347 = Wait (ms)(milliseconds to wait=u32 1000) -> ()  [unwired: 1 out]
          }
          frame #11 {
            n348 = property on="Fish for Tether" class="Bool (strict)"("Val(Sgnl)"=TRUE ("Value (Signaling)")) -> ()  [unwired: 2 in, 2 out]
          }
        }
        n349 = local write "Cal/Data Acq. Spot"(FALSE ("Cal/Data Acq. Spot")) -> ()
      }
      event "Dump Beads": Value Change {
        n350 = event-data() -> ()  [unwired: 1 in, 5 out]
        n351 = flat-sequence {
          tunnel: ["Dump spot flow on?"] -> w549
          tunnel: [w560] -> w550
          tunnel: w549 -> [w560]
          tunnel: w553 -> [w565]
          tunnel: w552 -> [w564]
          tunnel: [w562] -> w551
          tunnel: w550 -> [w562]
          tunnel: w551 -> [w575]
          frame #0 {
            n352 = local read "Saving..."() -> (w556:bool)
            n353 = local write "Dump Beads"(FALSE ("Dump Beads")) -> ()
            n354 = local write "Stop Saving"(w556) -> ()
          }
          frame #1 {
            w557 = FALSE ("Fl. Triggered...")
            n355 = case shown="True" "Dump spot flow on?" {
              frame False {
              }
              frame True {
                n356 = property on="Sample Channel\nFlow" class="Bool (strict)"("Val(Sgnl)"=TRUE ("Stage Moving")) -> ()  [unwired: 2 in, 2 out]
              }
            }
            n357 = local write "Fl. Triggered..."(w557) -> ()
            n358 = local write "Tether"(w557) -> ()
            n359 = property on="Green Laser ON/Interlacing" class="Bool (strict)"("Val(Sgnl)"=w557) -> ()  [unwired: 2 in, 2 out]
            n360 = property on="Trap Pos. FB ON" class="Bool (strict)"("Val(Sgnl)"=w557) -> ()  [unwired: 2 in, 2 out]
            n361 = property on="Trap Trig. Fl." class="Bool (strict)"("Val(Sgnl)"=w557) -> ()  [unwired: 2 in, 2 out]
            n362 = property on="Dip for Protein" class="Bool (strict)"("Val(Sgnl)"=w557) -> ()  [unwired: 2 in, 2 out]
            n363 = property on="Pause dwell \ntimer" class="Bool (strict)"("Val(Sgnl)"=w557) -> ()  [unwired: 2 in, 2 out]
          }
          frame #2 {
            n364 = property on="Trap Pos. FB Offset Factor" class="DigNum (strict)"("Val(Sgnl)"=i64 0 ("Value (Signaling)")) -> ()  [unwired: 2 in, 2 out]
          }
          frame #3 {
            n365 = local read "Saved Stage Positions"() -> (w566:dbl[][])
            n366 = local write "Stage Moving"(TRUE ("Stage Moving")) -> ()
            n367 = Array Subset(array=w566, index (row)=3 ("index"), length (row)=1 ("length"), index (col)=1 ("index"), length (col)=3 ("length")) -> (w571:dbl[][])
            n368 = Reshape Array(w571, 3 ("dimension size")) -> (w569:dbl[])
            n369 = Array To Cluster(array=w569) -> (cluster=w568:cluster{"[0]":dbl, "[1]":dbl, "[2]":dbl})
            n370 = call "Set Stage Position.vi"("Position"=w568, "error in"=w564, "VISA resource name in"=w565) -> ()  [unwired: 3 out]
          }
          frame #4 {
            w576 = FALSE ("Value (Signaling)")
            n371 = case shown="True" w575 {
              frame False {
              }
              frame True {
                n372 = property on="Sample Channel\nFlow" class="Bool (strict)"("Val(Sgnl)"=FALSE ("Stage Moving")) -> ()  [unwired: 2 in, 2 out]
              }
            }
            n373 = property on="Trap 1 (ON/OFF)" class="Bool (strict)"("Val(Sgnl)"=w576) -> ()  [unwired: 2 in, 2 out]
            n374 = property on="Trap 2 (ON/OFF)" class="Bool (strict)"("Val(Sgnl)"=w576) -> ()  [unwired: 2 in, 2 out]
            n375 = call <vilib>:"Beep.vi"() -> ()  [unwired: 3 in, 9 out]
          }
          frame #5 {
            n376 = property on="Move Cap. 2 (ADig Top)" class="Bool (strict)"("Val(Sgnl)"=TRUE ("Value (Signaling)")) -> ()  [unwired: 2 in, 2 out]
            n377 = property on="Tab Control" class="TabCtl (strict)"("Val(Sgnl)"=T4."Status" ("Value (Signaling)")) -> ()  [unwired: 2 in, 2 out]
          }
        }
      }
      event "Dip for Protein": Value Change {
        n378 = event-data() -> ()  [unwired: 1 in, 5 out]
        n379 = case shown="True" "Dip for Protein" {
          tunnel: w582 -> [_ w584]
          tunnel: w581 -> [_ w583]
          frame False {
          }
          frame True {
            n380 = while {
              tunnel: w584 -> [w592]
              tunnel: w583 -> [w591]
              i -> [w586]
              stop <- w588 stop-if-true
              n381 = Increment(x=w586) -> (x+1=→"Dip #":i32)
              n382 = flat-sequence {
                tunnel: w591 -> [w600]
                tunnel: w592 -> [w601]
                tunnel: [w601] -> w596
                tunnel: [w600] -> w595
                tunnel: [w604] -> w590
                tunnel: [w605] -> w589
                tunnel: w596 -> [w606]
                tunnel: w595 -> [w607]
                tunnel: [w614] -> w594
                tunnel: w590 -> [w614]
                tunnel: [w613] -> w593
                tunnel: w589 -> [w613]
                tunnel: [w610] -> w587
                tunnel: w593 -> [w634]
                tunnel: w594 -> [w635]
                tunnel: w587 -> [w636]
                tunnel: [w672] -> w588
                frame #0 {
                  n383 = case shown="True" "Move trap \nbefore dip move?" {
                    frame False {
                    }
                    frame True {
                      n384 = property on="Trap Delta (MHz)" class="DigNum (strict)"("Val(Sgnl)"="Dipping Delta (MHz)") -> ()  [unwired: 2 in, 2 out]
                    }
                  }
                  n385 = property on="Green Laser ON/Interlacing" class="Bool (strict)"("Val(Sgnl)"="Green ON\nbefore dip?") -> ()  [unwired: 2 in, 2 out]
                  n386 = property on="Sample Channel\nFlow" class="Bool (strict)"("Val(Sgnl)"="Flow ON\nduring dip?") -> ()  [unwired: 2 in, 2 out]
                }
                frame #1 {
                  n387 = local read "Saved Stage Positions"() -> (w609:dbl[][])
                  n388 = local write "Cancel dwell"(FALSE ("Cancel dwell")) -> ()
                  n389 = call "move to saved stage position.vi"("error in"=w607, "Stage VISA resource name in"=w606, "Position"="Dip Stage \nPosition", "Saved Stage Positions"=w609) -> ("VISA resource name out"=w604:refnum<visa-resource-name>, "error out"=w605:errorcluster)
                }
                frame #2 {
                  n390 = node-c288() -> (w612:T21)  [unwired: 4 in]
                  n391 = timed-loop {
                    timing: w612 -> [_]
                    timing-out: [_] -> w611
                    tunnel: [w618] -> w610
                    i -> [w629]
                    stop <- w619 stop-if-true
                    n392 = node-c288() -> ()  [unwired: 1 in, 1 out]
                    n393 = Increment(x=w629) -> (x+1=→"Dip Time (s)":i32)
                    n394 = Greater Or Equal?(x=w629, y="Dip Duration (s)") -> (x >= y?=w627:bool)
                    n395 = local read "Dip for Protein"() -> (w620:bool)
                    n396 = local read "Dump Beads"() -> (w617:bool)
                    n397 = local read "Cancel dwell"() -> (w626:bool)
                    n398 = local read "Pause dwell \ntimer"() -> (w623:bool)
                    n399 = Not(x=w620) -> (.not. x?=w625:bool)
